vi "UBX Message Response.vi"(8 "error in":errorcluster, 9 "Timeout (1000 ms)":u32=1000, 11 "VISA resource name":refnum<visa-resource-name>) -> (0 "error out":errorcluster, 2 "Message Acknowledged":bool, 3 "VISA resource name out":refnum<visa-resource-name>)   [LabVIEW 2009]
doc: "Checks to see if a sent UBX message has been acknowledged or not. See the UBX Protocol Specifications for more details."
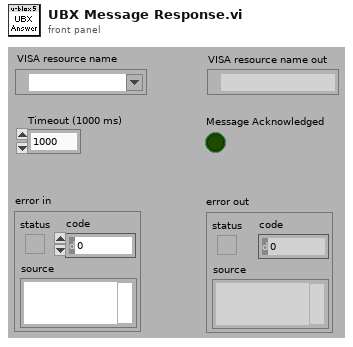
[diagram p1: front panel]
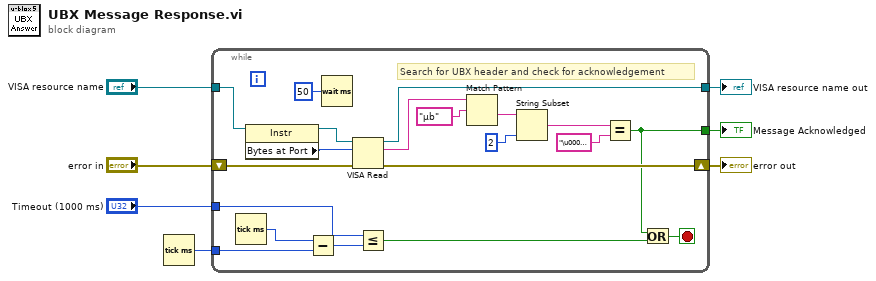
[diagram p0: block diagram]
diagram:
  n1 = Tick Count (ms)() -> (millisecond timer value=w4:u32)
  n2 = while {
    tunnel: "VISA resource name" -> [w19]
    tunnel: [w20] -> w1
    tunnel: w4 -> [w27]
    tunnel: "Timeout (1000 ms)" -> [w21]
    shift-right: [w14] -> w5
    shift-left: "error in" -> [w22]
    tunnel: [w9] -> w2
    stop <- w25 stop-if-true
    # "Search for UBX header and check for acknowledgement"
    n3 = Tick Count (ms)() -> (millisecond timer value=w26:u32)
    n4 = property class="Instr"(reference=w19) -> (reference out=w18:refnum<visa-resource-name>, "Bytes at Port"=w17:u32)  [unwired: 1 in, 1 out]
    n5 = Subtract(x=w26, y=w27) -> (x-y=w24:u32)
    n6 = Wait (ms)(milliseconds to wait=u32 50) -> ()  [unwired: 1 out]
    n7 = VISA Read(VISA resource name=w18, byte count=w17, error in (no error)=w22) -> (VISA resource name out=w20:refnum<visa-resource-name>, read buffer=w15:string, error out=w14:errorcluster)  [unwired: 1 out]
    n8 = Less Or Equal?(x=w21, y=w24) -> (x <= y?=w23:bool)
    n9 = Match Pattern(string=w15, regular expression="µb") -> (after substring=w10:string)  [unwired: 1 in, 3 out]
    n10 = String Subset(string=w10, length (rest)=2 ("length (rest)")) -> (substring=w12:string)  [unwired: 1 in]
    n11 = Equal?(x=w12, y="\u0005\u0001") -> (x = y?=w9:bool)
    n12 = Or(x=w9, y=w23) -> (x .or. y?=w25:bool)
  }
  "error out" <- w5
  "Message Acknowledged" <- w2
  "VISA resource name out" <- w1
